vi "Wfm Data FG.vi"(7 "Operation":enum16{"Initialize", "Reset", "Set", "Get"}(ring), 8 "Error In":errorcluster, 9 "Requested Buffer Size":dbl, 10 "Data Properties In":T1[](array[typedef]), 11 "New Data in":dbl[][](array[numeric])) -> (0 "Error Out":errorcluster, 2 "Data Properties dup":T1[](array[typedef]), 3 "Requested Data out":dbl[][](array[numeric]))   [LabVIEW 2014, in "Waveform-Processing-Custom-Device Engine.lvlib"]
uses:
  Waveform-Processing-Custom-Device Engine.lvlib
  <vilib>/NI Veristand/Custom Device Waveform API/Waveform properties.ctl
  <vilib>/NI Veristand/Custom Device API/Waveform Data Reference.ctl
  <vilib>/NI Veristand/Custom Device API/Custom Device API.lvlib
  <vilib>/NI Veristand/Custom Device Waveform API/NI_VS Custom Device Waveform API.lvlib
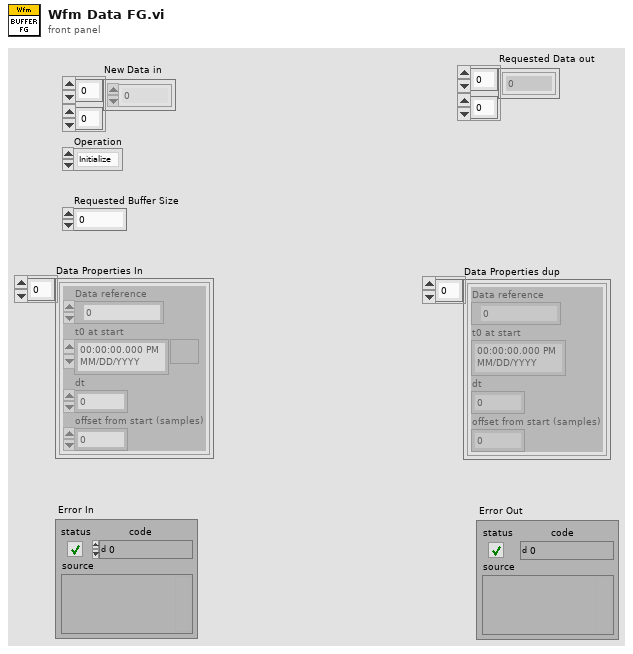
[diagram p1: front panel]
types:
  T1 = typedef "NI_VS Custom Device Waveform API.lvlib/Waveform properties.ctl" = cluster{"Data reference":T2, "t0 at start":timestamp, "dt":dbl, "offset from start (samples)":u64}
  T2 = typedef "Custom Device API.lvlib/Waveform Data Reference.ctl" = i32
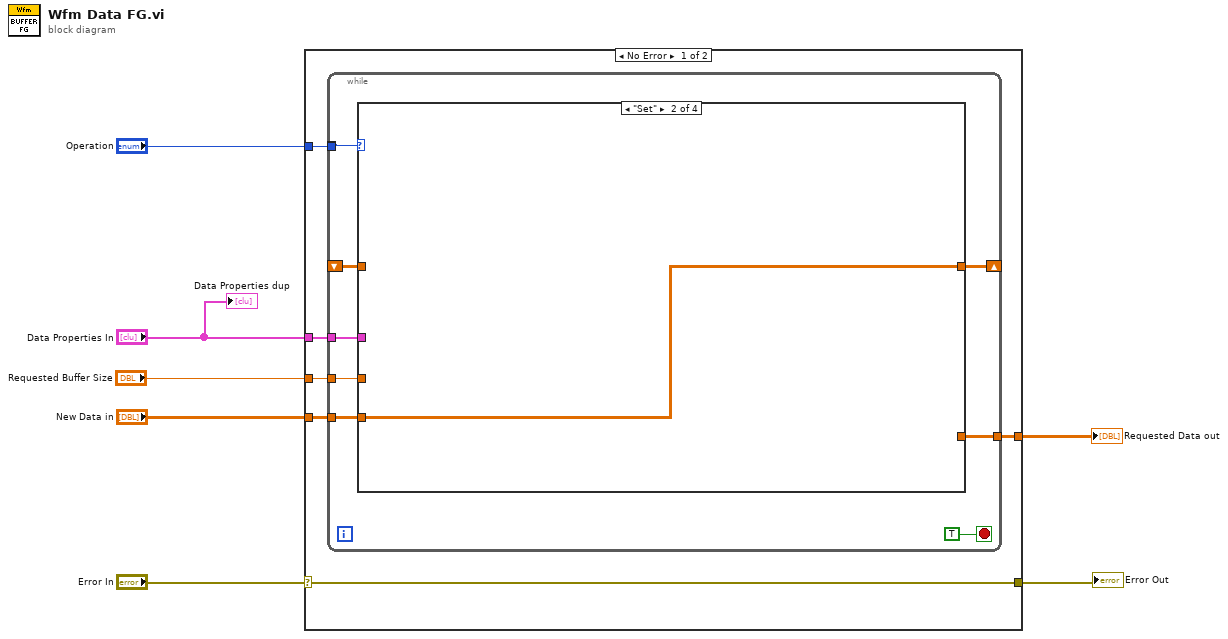
[diagram p0: block diagram]
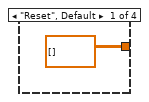
[diagram p2: hidden frame]
diagram:
  n1 = case shown="No Error" "Error In" {
    selector: "Error In" -> [w8 w26]
    tunnel: [w8 w26] -> w6
    tunnel: "Operation" -> [w13 _]
    tunnel: "Requested Buffer Size" -> [w12 _]
    tunnel: "Data Properties In" -> [w11 _]
    tunnel: "New Data in" -> [w10 _]
    tunnel: [w9 _] -> w2
    frame No Error {
      n2 = while {
        tunnel: [w20] -> _
        tunnel: w13 -> [w20]
        tunnel: w12 -> [w18]
        tunnel: w11 -> [w19]
        tunnel: w10 -> [w17]
        shift-right: [w15] -> _
        shift-left: _ -> [w16]
        tunnel: [w14] -> w9
        stop <- TRUE stop-if-true
        n3 = case shown="\"Set\"" w20 {
          tunnel: w19 -> [_ _ _ _]
          tunnel: w18 -> [_ _ _ _]
          tunnel: w17 -> [_ w23 _ _]
          tunnel: w16 -> [_ _ w24 w25]
          tunnel: [dbl[][] [] ("Requested Data out") w23 w24 w25] -> w15
          tunnel: [_ _ w24 _] -> w14
          frame "Reset", Default {
          }
          frame "Set" {
          }
          frame "Get" {
          }
          frame "Initialize" {
          }
        }
      }
    }
    frame Error {
    }
  }
  "Error Out" <- w6
  "Requested Data out" <- w2
  "Data Properties dup" <- "Data Properties In"
